vi "_Shift Rows Below Index.vi"(8 "error in":errorcluster, 10 "Row Index":i32, 11 "SheetData in":refnum<k24>) -> (0 "error out":errorcluster, 2 "Reference Row":refnum<k24>, 3 "SheetData out":refnum<k24>)   [LabVIEW 2021, in "Open Xml.lvlib"]
uses:
  Open Xml.lvlib
  D:/git/Open-Xml-LabVIEW/dll/DocumentFormat.OpenXml.dll
  dll/DocumentFormat.OpenXml.dll
  D:/git/Open-Xml-LabVIEW/dll/DocumentFormat.OpenXml.Framework.dll
  dll/DocumentFormat.OpenXml.Framework.dll
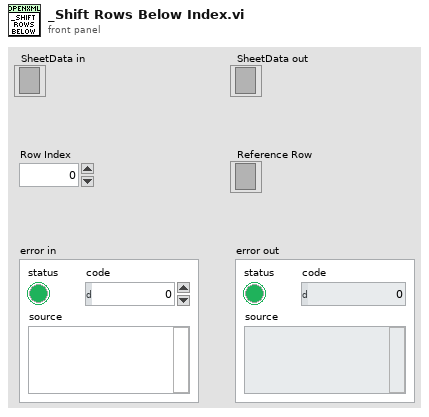
[diagram p1: front panel]
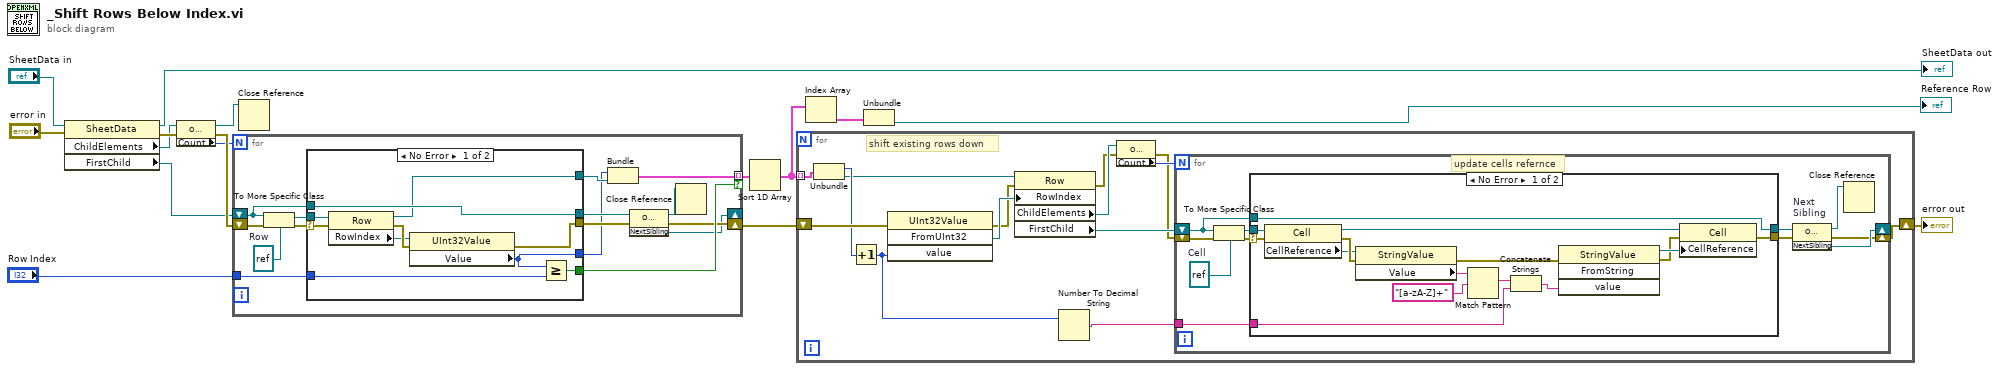
[diagram p0: block diagram]
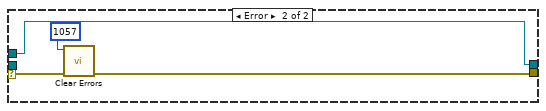
[diagram p2: hidden frame]
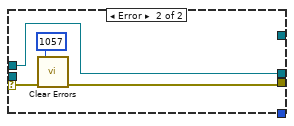
[diagram p3: hidden frame]
diagram:
  n1 = property class="SheetData"(reference="SheetData in", error in="error in") -> (reference out=→"SheetData out":refnum<k24>, error out=w9:errorcluster, "ChildElements"=w6:refnum<k24>, "FirstChild"=w8:refnum<k24>)
  n2 = property class="OpenXmlElementList"(reference=w6, error in=w9) -> (reference out=w11:refnum<k24>, error out=w10:errorcluster, "Count"=w7:i32)
  n3 = for {
    N: w7 -> [_]
    tunnel: "Row Index" -> [w27]
    tunnel: [w18] -> w12 mode=indexing if=w23
    shift-right: [w20] -> _
    shift-left: w8 -> [w25]
    shift-right: [w22] -> w13
    shift-left: w10 -> [w31]
    w30 = refnum<k24> refnum  # Row
    n4 = To More Specific Class(target class=w30, reference=w25, error in=w31) -> (specific class reference=w28:refnum<k24>, error out=w29:errorcluster)
    n5 = case shown="No Error" w29 {
      selector: w29 -> [w41 w44]
      tunnel: w28 -> [w40 _]
      tunnel: w27 -> [w34 _]
      tunnel: [w32 _] -> w26
      tunnel: [w37 _] -> w23
      tunnel: w25 -> [w36 w42]
      tunnel: [w35 w43] -> w24
      tunnel: [w36 w42] -> w21
      tunnel: [w33 _] -> w17
      frame No Error {
        n6 = property class="Row"(reference=w40, error in=w41) -> (reference out=w32:refnum<k24>, error out=w39:errorcluster, "RowIndex"=w38:refnum<k24>)
        n7 = property class="UInt32Value"(reference=w38, error in=w39) -> (error out=w35:errorcluster, "Value"=w33:u32)  [unwired: 1 out]
        n8 = Greater Or Equal?(x=w33, y=w34) -> (x >= y?=w37:bool)
      }
      frame Error {
        n9 = call <vilib>:"Clear Errors.vi"("error in (no error)"=w44, "specific error code to clear (0: all)"=1057) -> ("error out"=w43:errorcluster)  [unwired: 4 in, 1 out]
      }
    }
    n10 = Bundle("Value"=w17, "Row"=w26) -> (w18:cluster{"Value":u32, "Row":refnum<k24>})  [unwired: 1 in]
    n11 = invoke class="OpenXmlElement" method="NextSibling"(reference=w21, error in=w24) -> (reference out=w19:refnum<k24>, error out=w22:errorcluster, "NextSibling"=w20:refnum<k24>)  [unwired: 1 in]
    n12 = Close Reference(reference=w19) -> ()  [unwired: 1 in, 1 out]
  }
  n13 = Close Reference(reference=w11) -> ()  [unwired: 1 in, 1 out]
  n14 = Sort 1D Array(array=w12) -> (sorted array=w3:cluster{"Value":u32, "Row":refnum<k24>}[])
  n15 = for {
    tunnel: w3 -> [w59] mode=indexing
    shift-right: [w49] -> w16
    shift-left: w13 -> [w58]
    # "shift existing rows down"
    n16 = Unbundle(w59) -> ("Value"=w47:u32, "Row"=w46:refnum<k24>)
    n17 = Increment(x=w47) -> (x+1=w48:u32)
    n18 = invoke class="UInt32Value" method="FromUInt32"(error in=w58, "value"=w48) -> (error out=w55:errorcluster, "FromUInt32"=w57:refnum<k24>)  [unwired: 2 in, 2 out]
    n19 = property class="Row"(reference=w46, error in=w55, "RowIndex"=w57) -> (error out=w53:errorcluster, "ChildElements"=w54:refnum<k24>, "FirstChild"=w52:refnum<k24>)  [unwired: 1 out]
    n20 = Number To Decimal String(number=w48) -> (decimal integer string=w50:string)  [unwired: 1 in]
    n21 = property class="OpenXmlElementList"(reference=w54, error in=w53) -> (error out=w51:errorcluster, "Count"=w56:i32)  [unwired: 1 out]
    n22 = for {
      N: w56 -> [_]
      shift-right: [w61] -> w49
      shift-left: w51 -> [w69]
      tunnel: w50 -> [w65]
      shift-right: [w62] -> _
      shift-left: w52 -> [w64]
      w70 = refnum<k24> refnum  # Cell
      # "update cells refernce"
      n23 = To More Specific Class(target class=w70, reference=w64, error in=w69) -> (specific class reference=w67:refnum<k24>, error out=w68:errorcluster)
      n24 = case shown="No Error" w68 {
        selector: w68 -> [w85 w89]
        tunnel: w67 -> [w84 _]
        tunnel: [w73 w87] -> w66
        tunnel: w65 -> [w72 _]
        tunnel: w64 -> [w71 w86]
        tunnel: [w71 w86] -> w63
        frame No Error {
          n25 = property class="Cell"(reference=w84, error in=w85) -> (reference out=w79:refnum<k24>, error out=w83:errorcluster, "CellReference"=w82:refnum<k24>)
          n26 = property class="StringValue"(reference=w82, error in=w83) -> (error out=w75:errorcluster, "Value"=w81:string)  [unwired: 1 out]
          n27 = Match Pattern(string=w81, regular expression="[a-zA-Z]+") -> (match substring=w77:string)  [unwired: 1 in, 3 out]
          n28 = Concatenate Strings(w77, w72) -> (w76:string)
          n29 = invoke class="StringValue" method="FromString"(error in=w75, "value"=w76) -> (reference out=w78:refnum<k24>, error out=w74:errorcluster)  [unwired: 2 in, 2 out]
          n30 = property class="Cell"(reference=w79, error in=w74, "CellReference"=w78) -> (error out=w73:errorcluster)  [unwired: 1 out]
        }
        frame Error {
          n31 = call <vilib>:"Clear Errors.vi"("error in (no error)"=w89, "specific error code to clear (0: all)"=1057) -> ("error out"=w87:errorcluster)  [unwired: 4 in, 1 out]
        }
      }
      n32 = invoke on="Next\nSibling" class="OpenXmlElement" method="NextSibling"(reference=w63, error in=w66) -> (reference out=w60:refnum<k24>, error out=w61:errorcluster, "NextSibling"=w62:refnum<k24>)  [unwired: 1 in]
      n33 = Close Reference(reference=w60) -> ()  [unwired: 1 in, 1 out]
    }
  }
  "error out" <- w16
  n34 = Index Array(array=w3) -> (element=w2:cluster{"Value":u32, "Row":refnum<k24>})  [unwired: 1 in]
  n35 = Unbundle(w2) -> ("Row"=→"Reference Row":refnum<k24>)  [unwired: 1 out]
